vi "Keep largest (SubVI).vi"(9 "Reset":bool, 11 "Input":i32) -> (3 "Biggest":i32)   [LabVIEW 2013]
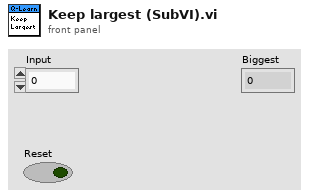
[diagram p1: front panel]
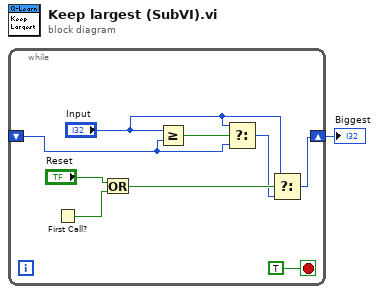
[diagram p0: block diagram]
diagram:
  n1 = while {
    shift-right: [w3] -> w1
    shift-left: _ -> [w8]
    stop <- TRUE stop-if-true
    n2 = First Call?() -> (First Call?: T/F=w6:bool)
    n3 = Or(x="Reset", y=w6) -> (x .or. y?=w5:bool)
    n4 = Greater Or Equal?(x="Input", y=w8) -> (x >= y?=w10:bool)
    n5 = Select(t="Input", s=w10, f=w8) -> (s? t:f=w4:i32)
    n6 = Select(t="Input", s=w5, f=w4) -> (s? t:f=w3:i32)
  }
  "Biggest" <- w1
